vi "Translate XBox Data.vi"(0 "Steer Axis":i32, 1 "Drive Axis":dbl, 8 "Limit Count Range":dbl=900000.0, 27 "Disable XBOX?":bool) -> (9 "Filtered Steer Axis":i32, 11 "Steer Counts":dbl, 13 "Filtered Drive Axis":dbl, 15 "Drive Voltage":dbl, 17 "Steer Value Output String":string, 19 "Drive Value Output String":string, 20 "Steer Value Output Number":dbl, 21 "Drive Value Output Number":dbl)   [LabVIEW 2011]
uses:
  <vilib>/express/express arith-compare/Formula/XNode/ExpressFormulaBlockNode.xnode
panel:
  in  "Drive (Keyboard Value)":dbl
  in  "Steer (Keyboard Value)":dbl
  in  "Over ride joystick":bool
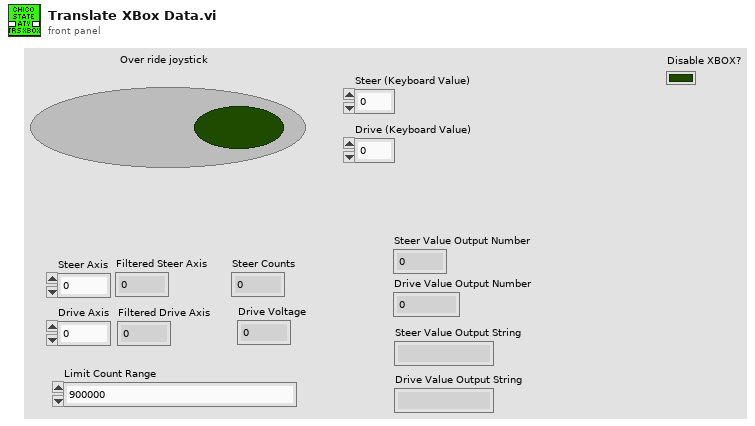
[diagram p1: front panel]
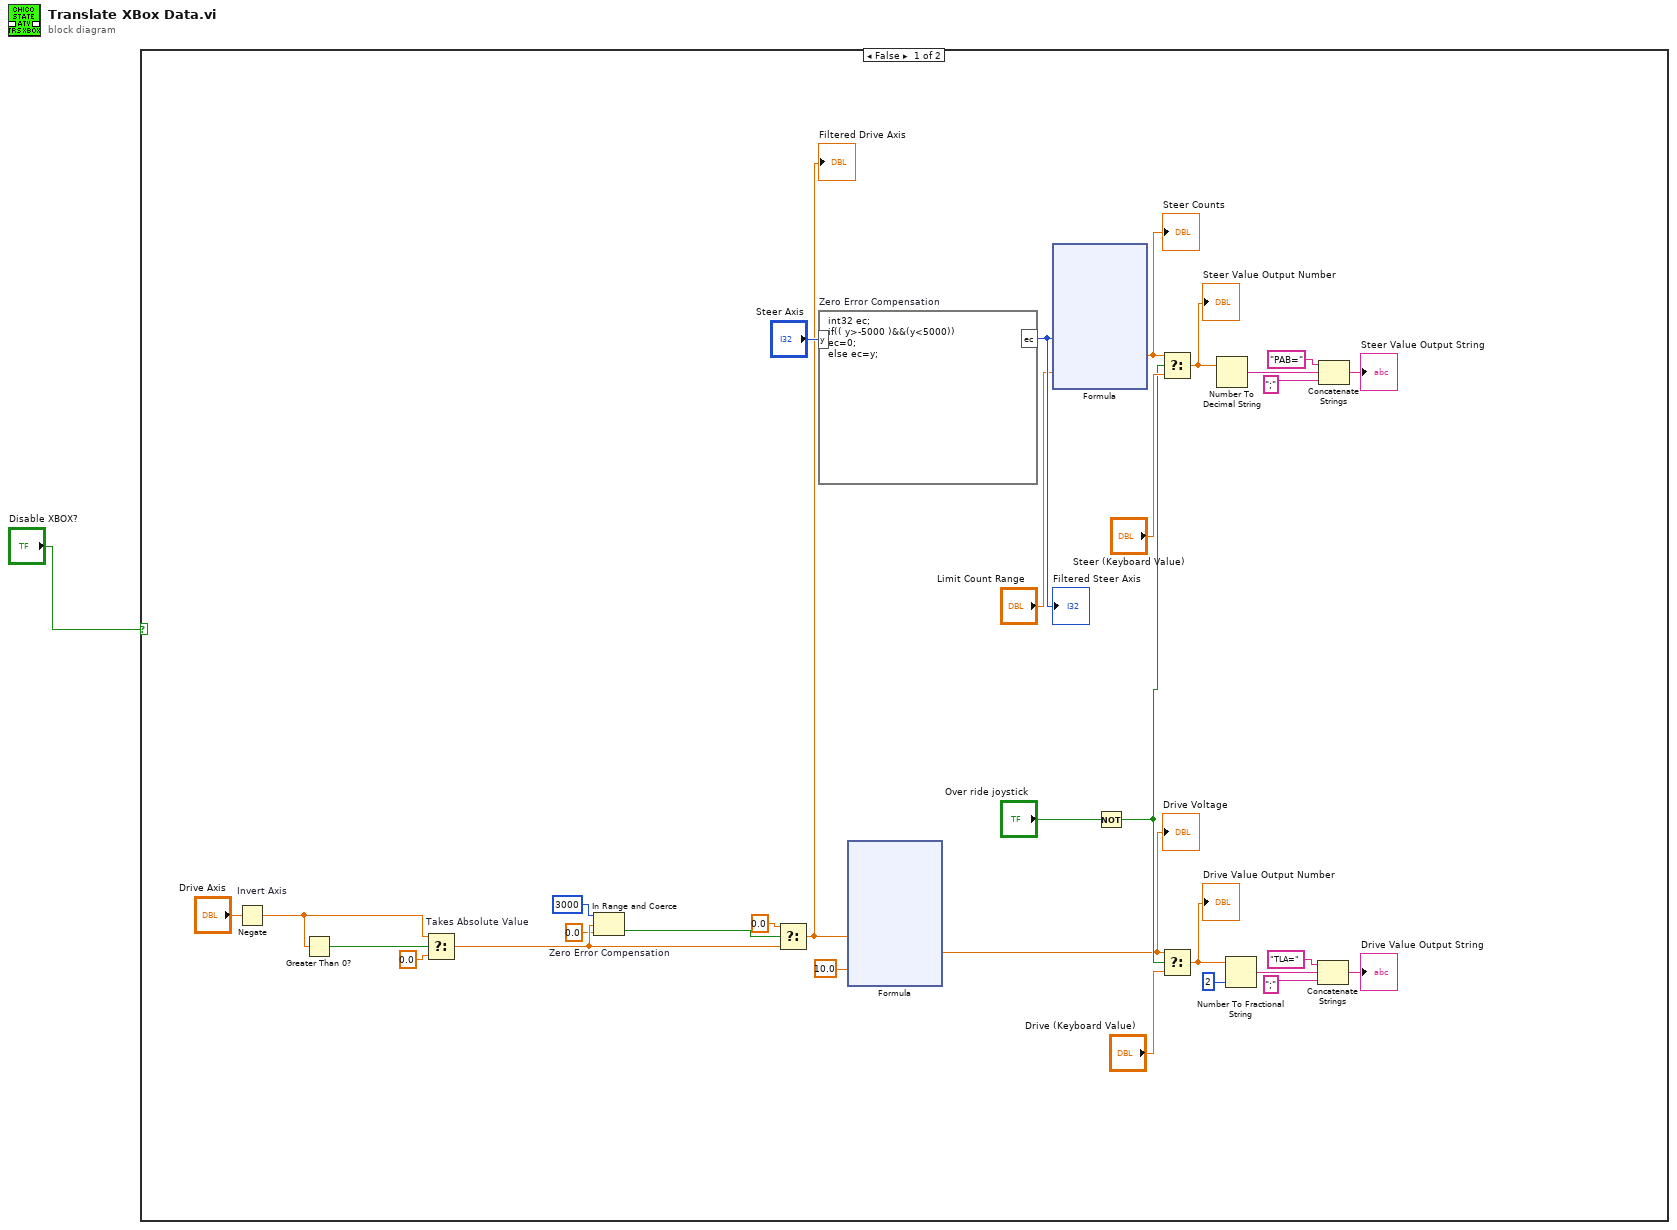
[diagram p0: block diagram]
diagram:
  n1 = case shown="False" "Disable XBOX?" {
    frame False {
      n2 = Negate "Invert Axis"(x="Drive Axis") -> (-x=w31:dbl)
      n3 = Greater Than 0?(x=w31) -> (x > 0?=w32:bool)
      n4 = Select "Takes Absolute Value"(t=w31, s=w32, f=0.0) -> (s? t:f=w28:dbl)
      n5 = In Range and Coerce "Zero Error Compensation"(upper limit=3000, x=w28, lower limit=0.0) -> (In Range?=w29:bool)  [unwired: 1 out]
      n6 = Select(t=0.0, s=w29, f=w28) -> (s? t:f=w14:dbl)
      "Filtered Drive Axis" <- w14
      n7 = formula code="int32 ec;\nif(( y>-5000 )&&(y<5000))\nec=0;\nelse ec=y;" "Zero Error Compensation"("y"="Steer Axis") -> ("ec"=w16:i32)
      "Filtered Steer Axis" <- w16
      n8 = xnode "Formula"("X1"=w14, "X2"=10.0) -> ("Result"=w13:dbl)  [unwired: 1 in, 1 out]
      "Drive Voltage" <- w13
      n9 = xnode "Formula"("X1"=w16, "X2"="Limit Count Range") -> ("Result"=w15:dbl)  [unwired: 1 in, 1 out]
      "Steer Counts" <- w15
      n10 = Not(x="Over ride joystick") -> (.not. x?=w21:bool)
      n11 = Select(t=w15, s=w21, f="Steer (Keyboard Value)") -> (s? t:f=w23:dbl)
      "Steer Value Output Number" <- w23
      n12 = Select(t=w13, s=w21, f="Drive (Keyboard Value)") -> (s? t:f=w24:dbl)
      "Drive Value Output Number" <- w24
      n13 = Number To Decimal String(number=w23) -> (decimal integer string=w5:string)  [unwired: 1 in]
      n14 = Number To Fractional String(number=w24, precision (6)=i16 2) -> (F-format string=w3:string)  [unwired: 2 in]
      n15 = Concatenate Strings("TLA=" ("string"), w3, ";" ("string")) -> (→"Drive Value Output String":string)
      n16 = Concatenate Strings("PAB=" ("string"), w5, ";" ("string")) -> (→"Steer Value Output String":string)
    }
    frame True {
    }
  }
